vi "AdquisicioDadesSAE.vi"(8 "Stop":refnum<vi>, 10 "user event":refnum<user-event>) -> ()   [LabVIEW 2017]
uses:
  <vilib>/DAQmx/read.llb/DAQmx Read (Analog 2D DBL NChan NSamp).vi
  <vilib>/DAQmx/miscellaneous.llb/DAQmx Fill In Error Info.vi
  <resource>/objmgr/daqmx.rc
panel:
  out "appended array":sgl[](array[numeric])
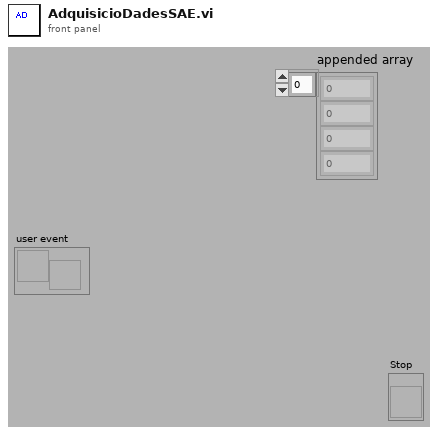
[diagram p1: front panel]
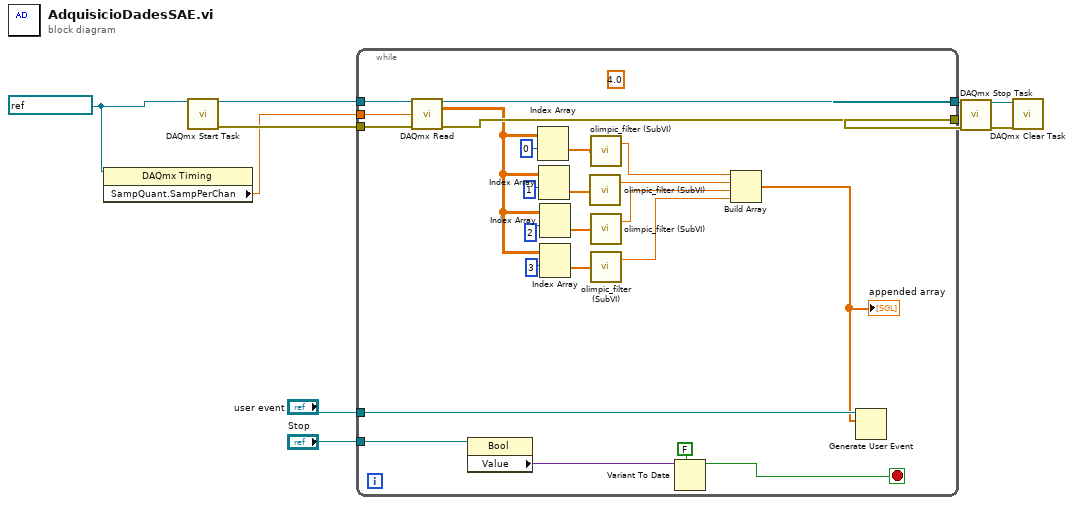
[diagram p0: block diagram]
diagram:
  w2 = refnum<k21> "SAE_Relats" ("task/channels in")
  n1 = property class="DAQmx Timing"(reference=w2) -> ("SampQuant.SampPerChan"=w1:dbl)  [unwired: 1 in, 2 out]
  n2 = call <vilib>:"DAQmx Start Task.vi"("task/channels in"=w2) -> ("task out"=w9:refnum<k21>, "error out"=w8:errorcluster)  [unwired: 13 in]
  n3 = while {
    tunnel: w9 -> [w26]
    tunnel: [w27] -> w10
    tunnel: w8 -> [w34]
    tunnel: "Stop" -> [w33]
    tunnel: [w30] -> w6
    tunnel: "user event" -> [w28]
    tunnel: w1 -> [w25]
    stop <- w29 stop-if-true
    (unwired) 4.0 ("Lower Cut-Off")
    n4 = call-poly <vilib>:"DAQmx Read.vi"("task/channels in"=w26, "number of samples per channel"=w25, "error in"=w34) -> ("task out"=w27:refnum<k21>, "data"=w17:dbl[][], "error out"=w30:errorcluster)  [unwired: 10 in]
    n5 = property class="Bool"(reference=w33) -> ("Value"=w32:variant)  [unwired: 1 in, 2 out]
    n6 = Index Array(array=w17, index (row)=0) -> (element=w12:dbl[])  [unwired: 1 in]
    n7 = Index Array(array=w17, index (row)=1) -> (element=w19:dbl[])  [unwired: 1 in]
    n8 = Index Array(array=w17, index (row)=2) -> (element=w18:dbl[])  [unwired: 1 in]
    n9 = Index Array(array=w17, index (row)=3) -> (element=w20:dbl[])  [unwired: 1 in]
    n10 = call "olimpic_filter (SubVI).vi"("array"=w19) -> ("olimpic_filter"=w16:sgl)  [unwired: 1 out]
    n11 = call "olimpic_filter (SubVI).vi"("array"=w12) -> ("olimpic_filter"=w11:sgl)  [unwired: 1 out]
    n12 = call "olimpic_filter (SubVI).vi"("array"=w18) -> ("olimpic_filter"=w15:sgl)  [unwired: 1 out]
    n13 = call "olimpic_filter (SubVI).vi"("array"=w20) -> ("olimpic_filter"=w14:sgl)  [unwired: 1 out]
    n14 = Variant To Data(type=FALSE, Variant=w32) -> (data=w29:bool)  [unwired: 1 in, 1 out]
    n15 = Build Array(w11, w16, w15, w14) -> (w13:sgl[])
    "appended array" <- w13
    n16 = Generate User Event(user event=w28, event data cluster=w13) -> ()  [unwired: 2 in, 2 out]
  }
  n17 = call <vilib>:"DAQmx Stop Task.vi"("task/channels in"=w10, "error in"=w6) -> ("task out"=w4:refnum<k21>, "error out"=w3:errorcluster)  [unwired: 12 in]
  n18 = call <vilib>:"DAQmx Clear Task.vi"("task in"=w4, "error in"=w3) -> ()  [unwired: 13 in, 1 out]
